vi "CRYGet Channel Calc Factor.vi"(4 "Signal Path":string, 6 "Channel Name":string, 7 "Audio Driver":u32, 8 "Is Input?":bool, 9 "I/O_channel Info":T4[](array[typedef]) {"Coupling" items=["Default"=-1, "RSE"=10083, "NRSE"=10078, "Differential"=10106, "Pseudodifferential"=12529]; "term config" items=["Default"=-1, "RSE"=10083, "NRSE"=10078, "Differential"=10106, "Pseudodifferential"=12529]; "Anti-aliasing Factor (%fs)" format="%.2f"}, 10 "Channel(LR)":u16, 11 "DeviceID":u32) -> (0 "Y unit":string, 1 "Calibration All Cluster":T1={"Calibration"={"Calibration Step Name"="", "Device"="", "Correction Curve Name"="", "Equalization Curve Name"="", "Sensitivity Curve Name"="", "Corr Folder and File"="", "EQ Folder and File"="", "Sens Folder and File"="", "Corr Step size"=0, "EQ Step size"=0, "Input"=FALSE, "Last Cal Date (sec)"=timestamp(0 s since 1904-01-01), "Cha Name"="", "Corr Curve Found"=FALSE, "EQ Curve Found"=FALSE, "Sens Curve Found"=FALSE, "Signal Type"="", "Calibrated Device"="", "Hz"=0}, "Corr Curve"={"Name"="", "Curve"=[], "X data"=1, "Y data"=1, "Z data"=1, "X axis"=0, "Y axis"=1, "Z axis"=1, "X unit"="", "Y unit"="", "Z unit"="deg.", "X dB ref"=1.0, "Y dB ref"=1.0, "Z dB ref"=1.0, "single val"=FALSE, "protected"=FALSE, "display X"=FALSE, "display Y"=TRUE, "display Z"=TRUE, "Test Info"="", "Step No."=0, "Plot Settings"={"Color"=0, "Interpolation"=0, "Point Style"=0, "Line Style"=0, "Point Color"=0, "Line Width"=0, "Bar Plot Style"=0, "Fill To"=0}, "AutoProtect"=FALSE}, "EQ Curve"={"Name"="", "Curve"=[], "X data"=1, "Y data"=1, "Z data"=1, "X axis"=0, "Y axis"=1, "Z axis"=1, "X unit"="Hz", "Y unit"="", "Z unit"="deg.", "X dB ref"=1.0, "Y dB ref"=1.0, "Z dB ref"=1.0, "single val"=FALSE, "protected"=FALSE, "display X"=TRUE, "display Y"=TRUE, "display Z"=TRUE, "Test Info"="", "Step No."=0, "Plot Settings"={"Color"=0, "Interpolation"=0, "Point Style"=0, "Line Style"=0, "Point Color"=0, "Line Width"=0, "Bar Plot Style"=0, "Fill To"=0}, "AutoProtect"=FALSE}, "Sens Curve"={"Name"="", "Curve"=[], "X data"=1, "Y data"=1, "Z data"=1, "X axis"=0, "Y axis"=1, "Z axis"=1, "X unit"="Hz", "Y unit"="", "Z unit"="deg.", "X dB ref"=1.0, "Y dB ref"=1.0, "Z dB ref"=1.0, "single val"=FALSE, "protected"=FALSE, "display X"=TRUE, "display Y"=TRUE, "display Z"=TRUE, "Test Info"="", "Step No."=0, "Plot Settings"={"Color"=0, "Interpolation"=0, "Point Style"=0, "Line Style"=0, "Point Color"=0, "Line Width"=0, "Bar Plot Style"=0, "Fill To"=0}, "AutoProtect"=FALSE}} {"Sens Curve"."Z data" items=["dB", "Lin"]; "Sens Curve"."X data" items=["dB", "Lin"]; "Sens Curve"."Y data" items=["dB", "Lin"]; "Sens Curve"."Z dB ref" format="%.1f"; "Sens Curve"."Z axis" items=["Log", "Lin"]; "Sens Curve"."X dB ref" format="%.1f"; "Sens Curve"."X axis" items=["Log", "Lin"]; "Sens Curve"."Y axis" items=["Log", "Lin"]; "Sens Curve"."Y dB ref" format="%.1f"; "Sens Curve"."Curve"."z" format="%.2f"; "Sens Curve"."Curve"."y" format="%.2f"; "Sens Curve"."Curve"."x" format="%.2f"; "EQ Curve"."Z data" items=["dB", "Lin"]; "EQ Curve"."X data" items=["dB", "Lin"]; "EQ Curve"."Y data" items=["dB", "Lin"]; "EQ Curve"."Z dB ref" format="%.1f"; "EQ Curve"."Z axis" items=["Log", "Lin"]; "EQ Curve"."X dB ref" format="%.1f"; "EQ Curve"."X axis" items=["Log", "Lin"]; "EQ Curve"."Y axis" items=["Log", "Lin"]; "EQ Curve"."Y dB ref" format="%.1f"; "EQ Curve"."Curve"."z" format="%.2f"; "EQ Curve"."Curve"."y" format="%.2f"; "EQ Curve"."Curve"."x" format="%.2f"; "Corr Curve"."Z data" items=["dB", "Lin"]; "Corr Curve"."X data" items=["dB", "Lin"]; "Corr Curve"."Y data" items=["dB", "Lin"]; "Corr Curve"."Z dB ref" format="%.1f"; "Corr Curve"."Z axis" items=["Log", "Lin"]; "Corr Curve"."X dB ref" format="%.1f"; "Corr Curve"."X axis" items=["Log", "Lin"]; "Corr Curve"."Y axis" items=["Log", "Lin"]; "Corr Curve"."Y dB ref" format="%.1f"; "Corr Curve"."Curve"."z" format="%.2f"; "Corr Curve"."Curve"."y" format="%.2f"; "Corr Curve"."Curve"."x" format="%.2f"; "Calibration"."EQ Step size" items=["R10", "R20", "R40", "R80", "User"]; "Calibration"."Corr Step size" items=["R10", "R20", "R40", "R80", "User"]}, 2 "Bit Max Level":dbl, 3 "Calc Factor":dbl)   [LabVIEW 2013]
uses:
  Typedef Control/CRYHardware Channel Info.ctl
  Typedef Control/CRYCalibration 2DCluster.ctl
  Typedef Control/CRYCalibration Cluster.ctl
  Typedef Control/CRYData Cluster.ctl
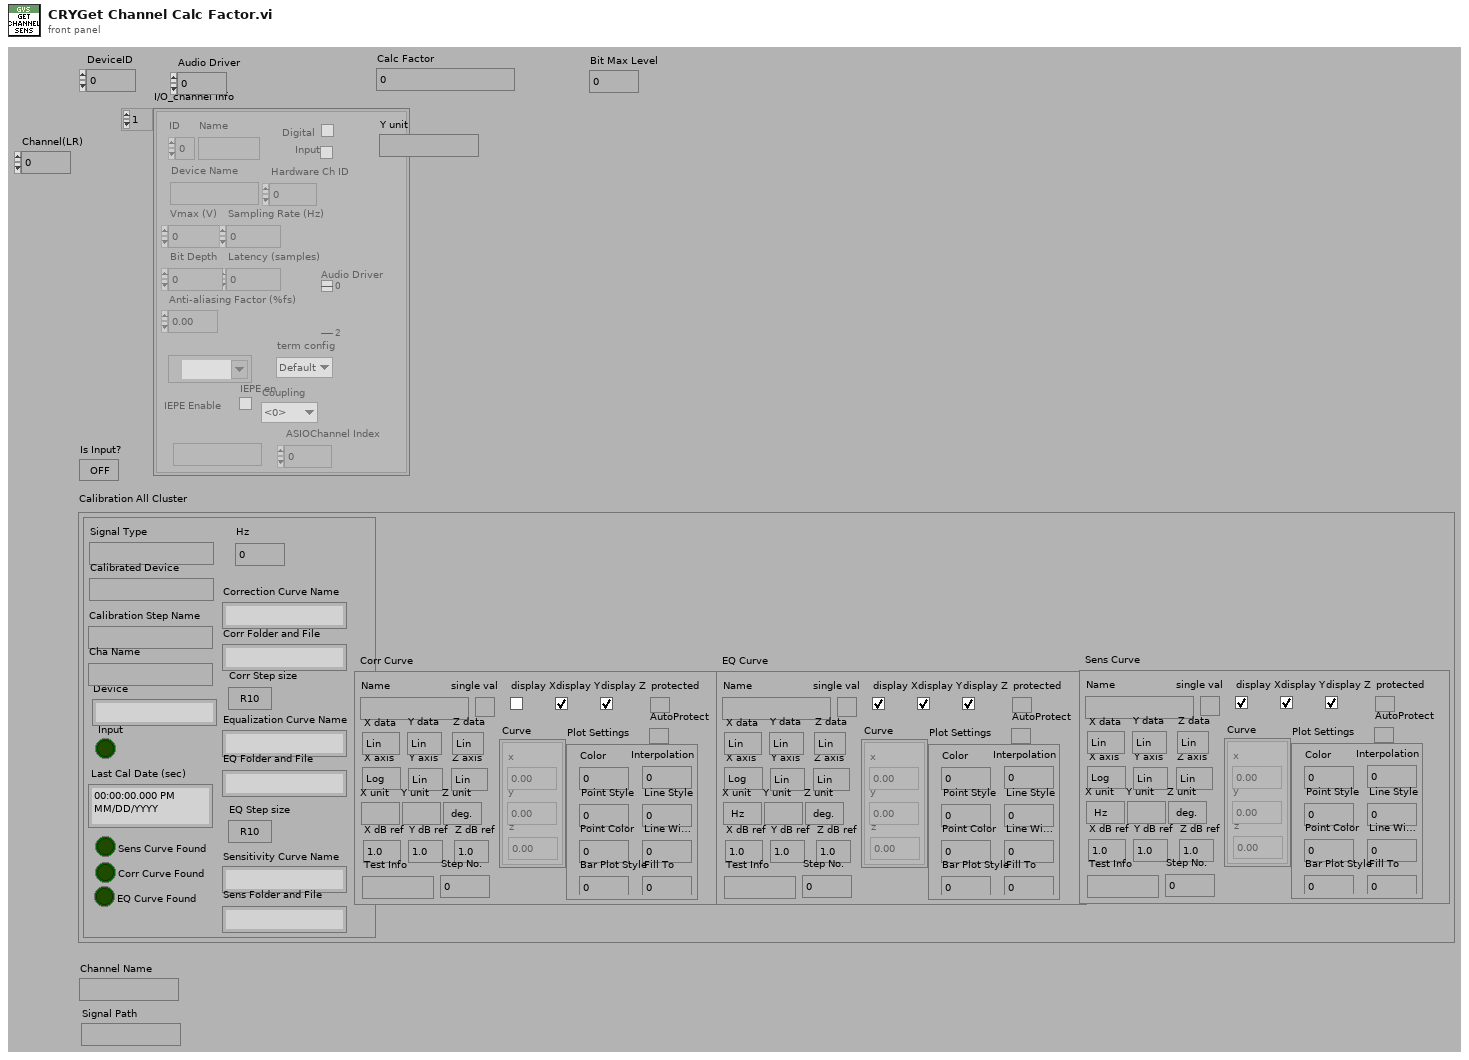
[diagram p1: front panel]
types:
  T1 = typedef "CRYCalibration 2DCluster.ctl" = cluster{"Calibration":T2, "Corr Curve":T3, "EQ Curve":T3, "Sens Curve":T3}
  T2 = typedef "CRYCalibration Cluster.ctl" = cluster{"Calibration Step Name":string, "Device":string, "Correction Curve Name":string, "Equalization Curve Name":string, "Sensitivity Curve Name":string, "Corr Folder and File":string, "EQ Folder and File":string, "Sens Folder and File":string, "Corr Step size":u16, "EQ Step size":u16, "Input":bool, "Last Cal Date (sec)":timestamp, "Cha Name":string, "Corr Curve Found":bool, "EQ Curve Found":bool, "Sens Curve Found":bool, "Signal Type":string, "Calibrated Device":string, "Hz":u32}
  T3 = typedef "CRYData Cluster.ctl" = cluster{"Name":string, "Curve":cluster{"x":dbl, "y":dbl, "z":dbl}[], "X data":u16, "Y data":u16, "Z data":u16, "X axis":u16, "Y axis":u16, "Z axis":u16, "X unit":string, "Y unit":string, "Z unit":string, "X dB ref":dbl, "Y dB ref":dbl, "Z dB ref":dbl, "single val":bool, "protected":bool, "display X":bool, "display Y":bool, "display Z":bool, "Test Info":string, "Step No.":i32, "Plot Settings":cluster{"Color":u32, "Interpolation":u8, "Point Style":u8, "Line Style":u8, "Point Color":u32, "Line Width":u8, "Bar Plot Style":u8, "Fill To":i16}, "AutoProtect":bool}
  T4 = typedef "CRYHardware Channel Info.ctl" = cluster{"ID":i32, "Name":string, "Digital":bool, "Input":bool, "Device Name":string, "Hardware Ch ID":u8, "Vmax (V)":dbl, "Latency (samples)":dbl, "Sampling Rate (Hz)":u32, "Bit Depth":u32, "Anti-aliasing Factor (%fs)":sgl, "DAQmx Channel":tag, "term config":i32, "Coupling":i32, "IEPE en":bool, "ASIOChannel Name":string, "Audio Driver":u16, "ASIOChannel Index":u8}
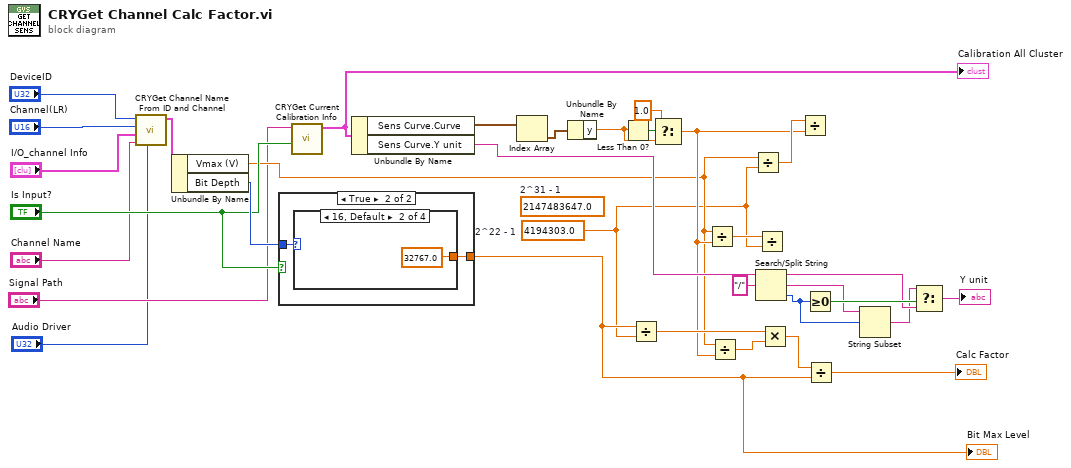
[diagram p0: block diagram]
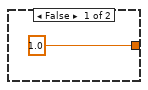
[diagram p2: hidden frame]
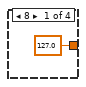
[diagram p3: hidden frame]
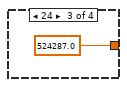
[diagram p4: hidden frame]
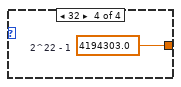
[diagram p5: hidden frame]
diagram:
  w3 = 4194303.0  # 2^22 - 1
  (unwired) 2147483647.0  # 2^31 - 1
  n1 = call "CRYGet Channel Name From ID and Channel.vi"("Audio Driver"="Audio Driver", "Channel Name"="Channel Name", "I/O_channel Info"="I/O_channel Info", "Channel(LR)"="Channel(LR)", "DeviceID"="DeviceID") -> ("Channel Info"=w24:T4)  [unwired: 6 out]
  n2 = Unbundle By Name(w24) -> ("Vmax (V)"=w7:dbl, "Bit Depth"=w13:u32)
  n3 = case shown="True" "Is Input?" {
    tunnel: w13 -> [_ w36]
    tunnel: [1.0 w35] -> w5
    frame False {
    }
    frame True {
      n4 = case shown="16, Default" w36 {
        tunnel: [127.0 ("2^31 - 1") 32767.0 524287.0 w40] -> w35
        frame 8 {
        }
        frame 16, Default {
        }
        frame 24 {
        }
        frame 32 {
          w40 = 4194303.0  # 2^22 - 1
        }
      }
    }
  }
  "Bit Max Level" <- w5
  n5 = call "CRYGet Current Calibration Info.vi"("Is Input?"="Is Input?", "Signal Type Name"="Signal Path") -> ("Calibration All Cluster"=w30:T1)  [unwired: 9 out]
  "Calibration All Cluster" <- w30
  n6 = Unbundle By Name(w30) -> ("Sens Curve.Curve"=w28:cluster{"x":dbl, "y":dbl, "z":dbl}[], "Sens Curve.Y unit"=w20:string)
  n7 = Index Array(array=w28) -> (element=w29:cluster{"x":dbl, "y":dbl, "z":dbl})  [unwired: 1 in]
  n8 = Unbundle By Name(w29) -> ("y"=w33:dbl)
  n9 = Less Than 0?(x=w33) -> (x < 0?=w31:bool)
  n10 = Divide(x=w5, y=w3) -> (x/y=w10:dbl)
  n11 = Select(t=1.0, s=w31, f=w33) -> (s? t:f=w8:dbl)
  n12 = Divide(x=w7, y=w8) -> (x/y=w14:dbl)
  n13 = Divide(x=w7, y=w8) -> (x/y=w11:dbl)
  n14 = Divide(x=w7, y=w3) -> (x/y=w15:dbl)
  n15 = Search/Split String(string=w20, search string/char (-)="/" ("search char (-)")) -> (substring before match=w21:string, match + rest of string=w18:string, offset of match=w17:i32)  [unwired: 1 out]
  n16 = Divide(x=w14, y=w3) -> ()  [unwired: 1 out]
  n17 = Multiply(x=w10, y=w11) -> (x*y=w9:dbl)
  n18 = Divide(x=w15, y=w8) -> ()  [unwired: 1 out]
  n19 = Greater Or Equal To 0?(x=w17) -> (x >= 0?=w22:bool)
  n20 = Divide(x=w9, y=w5) -> (x/y=→"Calc Factor":dbl)
  n21 = String Subset(string=w18, offset (0)=w17) -> (substring=w16:string)  [unwired: 1 in]
  n22 = Select(t=w16, s=w22, f=w21) -> (s? t:f=→"Y unit":string)
